vi "MC Control Loop.vi"() -> ()   [LabVIEW 2014]
uses:
  MC State Machine.lvsc/StatechartState.ctl
  MC State Machine.lvsc/State.ctl
  CAN Frame.ctl
  <vilib>/Platform/TimedLoop/XDataNode/timing_clust.ctl
  <vilib>/Platform/TimedLoop/XDataNode/nitl_modes.ctl
  <vilib>/Platform/TimedLoop/XDataNode/wakeup.ctl
  Remote Calibration/Remote Calibration Typedef.ctl
  MC State Machine.lvsc/Inputs.ctl
  AIR Status.ctl
  MC State Machine.lvsc/CompanionDiagram.vi/6/SC Main.vi
  CAN/8byte to 4 2byte.vi
  CAN/Decode VSM.vi
  CAN/Decode Inverter State.vi
  CAN/Decode Inverter Enable States.vi
  CAN/Decode Inverter Command Modes.vi
  CAN/MC/Process Run Fault.vi
  CAN/BMS/Decode Car State.vi
  CAN/BMS/Scale Cell Voltage.vi
  CAN/BMS/Scale Cell Temp.vi
  MC State Machine.lvsc/CompanionDiagram.vi/6/Upd State.vi
  MC State Machine.lvsc/CompanionDiagram.vi/6/Trans Graph0.vi
  MC State Machine.lvsc/CompanionDiagram.vi/6/EnterGraphCore.vi
  CAN/Send Throttle Signal.vi
  CAN/Disable Controller.vi
  CAN/MC/Clear Faults.vi
  CAN/Init Controller.vi
  CAN/MC/Send Parameter Message.vi
  <vilib>/FPGAPlugInAG/sbRIO-9626/niLvFpga_Open_sbRIO-9626.vi
  Global Data.vi
  <vilib>/Utility/error.llb/Error Cluster From Error Code.vi
  <vilib>/rvi/errors/niLvFpgaAdjustHostInterfaceError.vi
  MC State Machine.lvsc/CompanionDiagram.vi
  Percent to Torque Request.vi
  <vilib>/RioEmbeddedCAN/RioEmbeddedCAN.llb/CANWrite.vi
  <vilib>/FPGAPlugInAG/sbRIO-9626/niLvFpga_Close_sbRIO-9626.vi
  CAN/BMS/Decode Charging State.vi
  <vilib>/rvi/interface/nirviOpenFPGA/nirviOpenFPGA.xnode
  FPGA Bitfiles/FormulaElectric2_FPGATarget_FPGA_8a5J0mMac2U.lvbitx
  <vilib>/Platform/TimedLoop/XDataNode/XDataNode.xnode
  MC State Machine.lvsc/Trigger.ctl
  <vilib>/rvi/interface/nirviReadWriteControl/nirviReadWriteControl.xnode
  <vilib>/Statechart/Infrastructure/RTStatechart/RunTime SCN.xnode
  MC State Machine.lvsc/Outputs.ctl
  MC State Machine.lvsc
  <vilib>/rvi/interface/nirviCloseFPGA/nirviCloseFPGA.xnode
  <vilib>/Platform/TimedLoop/XDataNode/XDNodeRunTimeDep.lvlib
  NiFpgaLv.dll
panel:
  in  "Adjust Gamma Offset":bool
  in  "Gamma Adjust":dbl=120.0
  out "Active States":T1=[enum."Disabled"]
  in  "MC Update Period (ms)":u32=100
  in  "Zero Torque %":dbl
  in  "MC CAN Offset":u32=512 format="%x"
  in  "Regen Mult.":dbl
  in  "Torque Mult.":dbl=160.0
  in  "Activation Brake Pressure":dbl=50.0
  out "Torque Request":dbl=nan
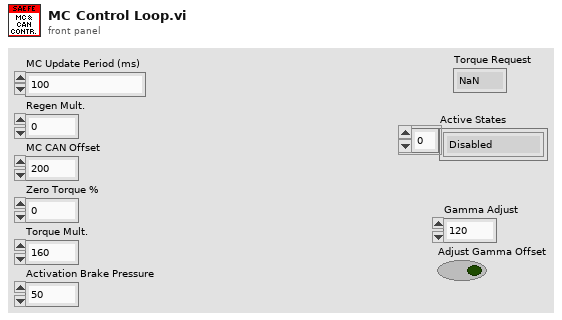
[diagram p1: front panel]
types:
  T1 = typedef "MC State Machine.lvsc/StatechartState.ctl" = T2[]
  T2 = typedef "MC State Machine.lvsc/State.ctl" = enum16{"NI.SC.Initial", "NI.SC.History", "NI.SC.ShallowHistory", "NI.SC.Terminal", "Let Current Drop then Disable AIR's", "Enabled", "Disabled"}
  T3 = typedef "CAN Frame.ctl" = cluster{"Time Stamp":timestamp, "Identifier":u32, "Extended":bool, "type":u8, "Payload":u8, "Payload 2":u8, "Payload 3":u8, "Payload 4":u8, "Payload 5":u8, "Payload 6":u8, "Payload 7":u8, "Payload 8":u8}
  T4 = cluster{"read mode":enum16{"polling", "blocking"}, "write mode":enum16{"polling", "blocking"}}
  T5 = typedef "Remote Calibration Typedef.ctl" = cluster{"Rear BP Scaling Factor":fxp<+,11,11>, "Front BP Scaling Factor":fxp<+,11,11>, "Rear BP Offset (V)":fxp<+/-,26,5>, "Front BP Offset":fxp<+/-,26,5>, "Throttle 2 Max":fxp<+,16,4>, "Throttle 2 Min":fxp<+,16,4>, "Throttle 1 Max":fxp<+,16,4>, "Throttle 1 Min":fxp<+,16,4>, "MC Update Period (ms)":u32, "Regen Mult.":dbl, "Zero Torque %":dbl, "Torque Mult.":dbl, "Activation Brake Pressure":dbl}
  T6 = typedef "XDNodeRunTimeDep.lvlib/timing_clust.ctl" = cluster{"Expected End [f-1]":u64, "Actual End [f-1]":u64, "Finished Late? [f-1]":bool, "Expected End [i-1]":u64, "Actual End [i-1]":u64, "Finished Late? [i-1]":bool, "Expected Start [i]":u64, "Actual Start [i]":u64, "Expected Start [f]":u64, "Actual Start [f]":u64, "Source Name":string, "Structure Name":string, "Period":i64, "Deadline":i64, "Offset":i64, "Start":i64, "Priority":i32, "Timeout":i32, "Mode":T7, "Wakeup Reason":T8, "Error":errorcluster, "Source Type":string, "Secondary Source Type":string, "Global End Time":u64, "Global Start Time":u64, "Frame Duration":u64, "Iteration Duration":u64, "Assigned CPU":i32, "I/O Scan Engine Mode":u32}
  T7 = typedef "XDNodeRunTimeDep.lvlib/nitl_modes.ctl" = enum32{"No Change", "Process missed periods, maintain original phase", "Discard missed periods, maintain original phase", "Process missed periods, ignore original phase", "Discard missed periods, ignore original phase"}
  T8 = typedef "XDNodeRunTimeDep.lvlib/wakeup.ctl" = enum32{"Normal", "Aborted", "Asynchronous wakeup", "Timing source error", "Timed loop error", "Timeout"}
  T9 = typedef "MC State Machine.lvsc/Inputs.ctl" = cluster{"Zero Torque %":dbl, "CAN Offset":u32, "Torque Mult.":dbl, "Regen Mult.":dbl, "Activation Brake Pressure":dbl, "stop":bool, "Average Throttle %":dbl, "Front Brake Pressure (psi)":dbl, "Motor Controller Dash Switch":bool, "Throttles OK?":bool, "AIR Status":T10, "CAN error":errorcluster, "CAN in":refnum<k20>, "tdms file":refnum<k34>, "tdms error":errorcluster, "Sampling Frequency (Hz)":dbl}
  T10 = typedef "AIR Status.ctl" = enum16{"Off", "Precharge", "On"}
  T11 = typedef "MC State Machine.lvsc/Outputs.ctl" = cluster{"Torque Request":dbl, "CAN error":errorcluster, "CAN out":refnum<k20>, "tdms file":refnum<k34>, "tdms error":errorcluster}
  T12 = typedef "CANFrameControl.ctl" = cluster{"identifier":u32, "extended?":bool, "type":u8, "payload":u8[]}
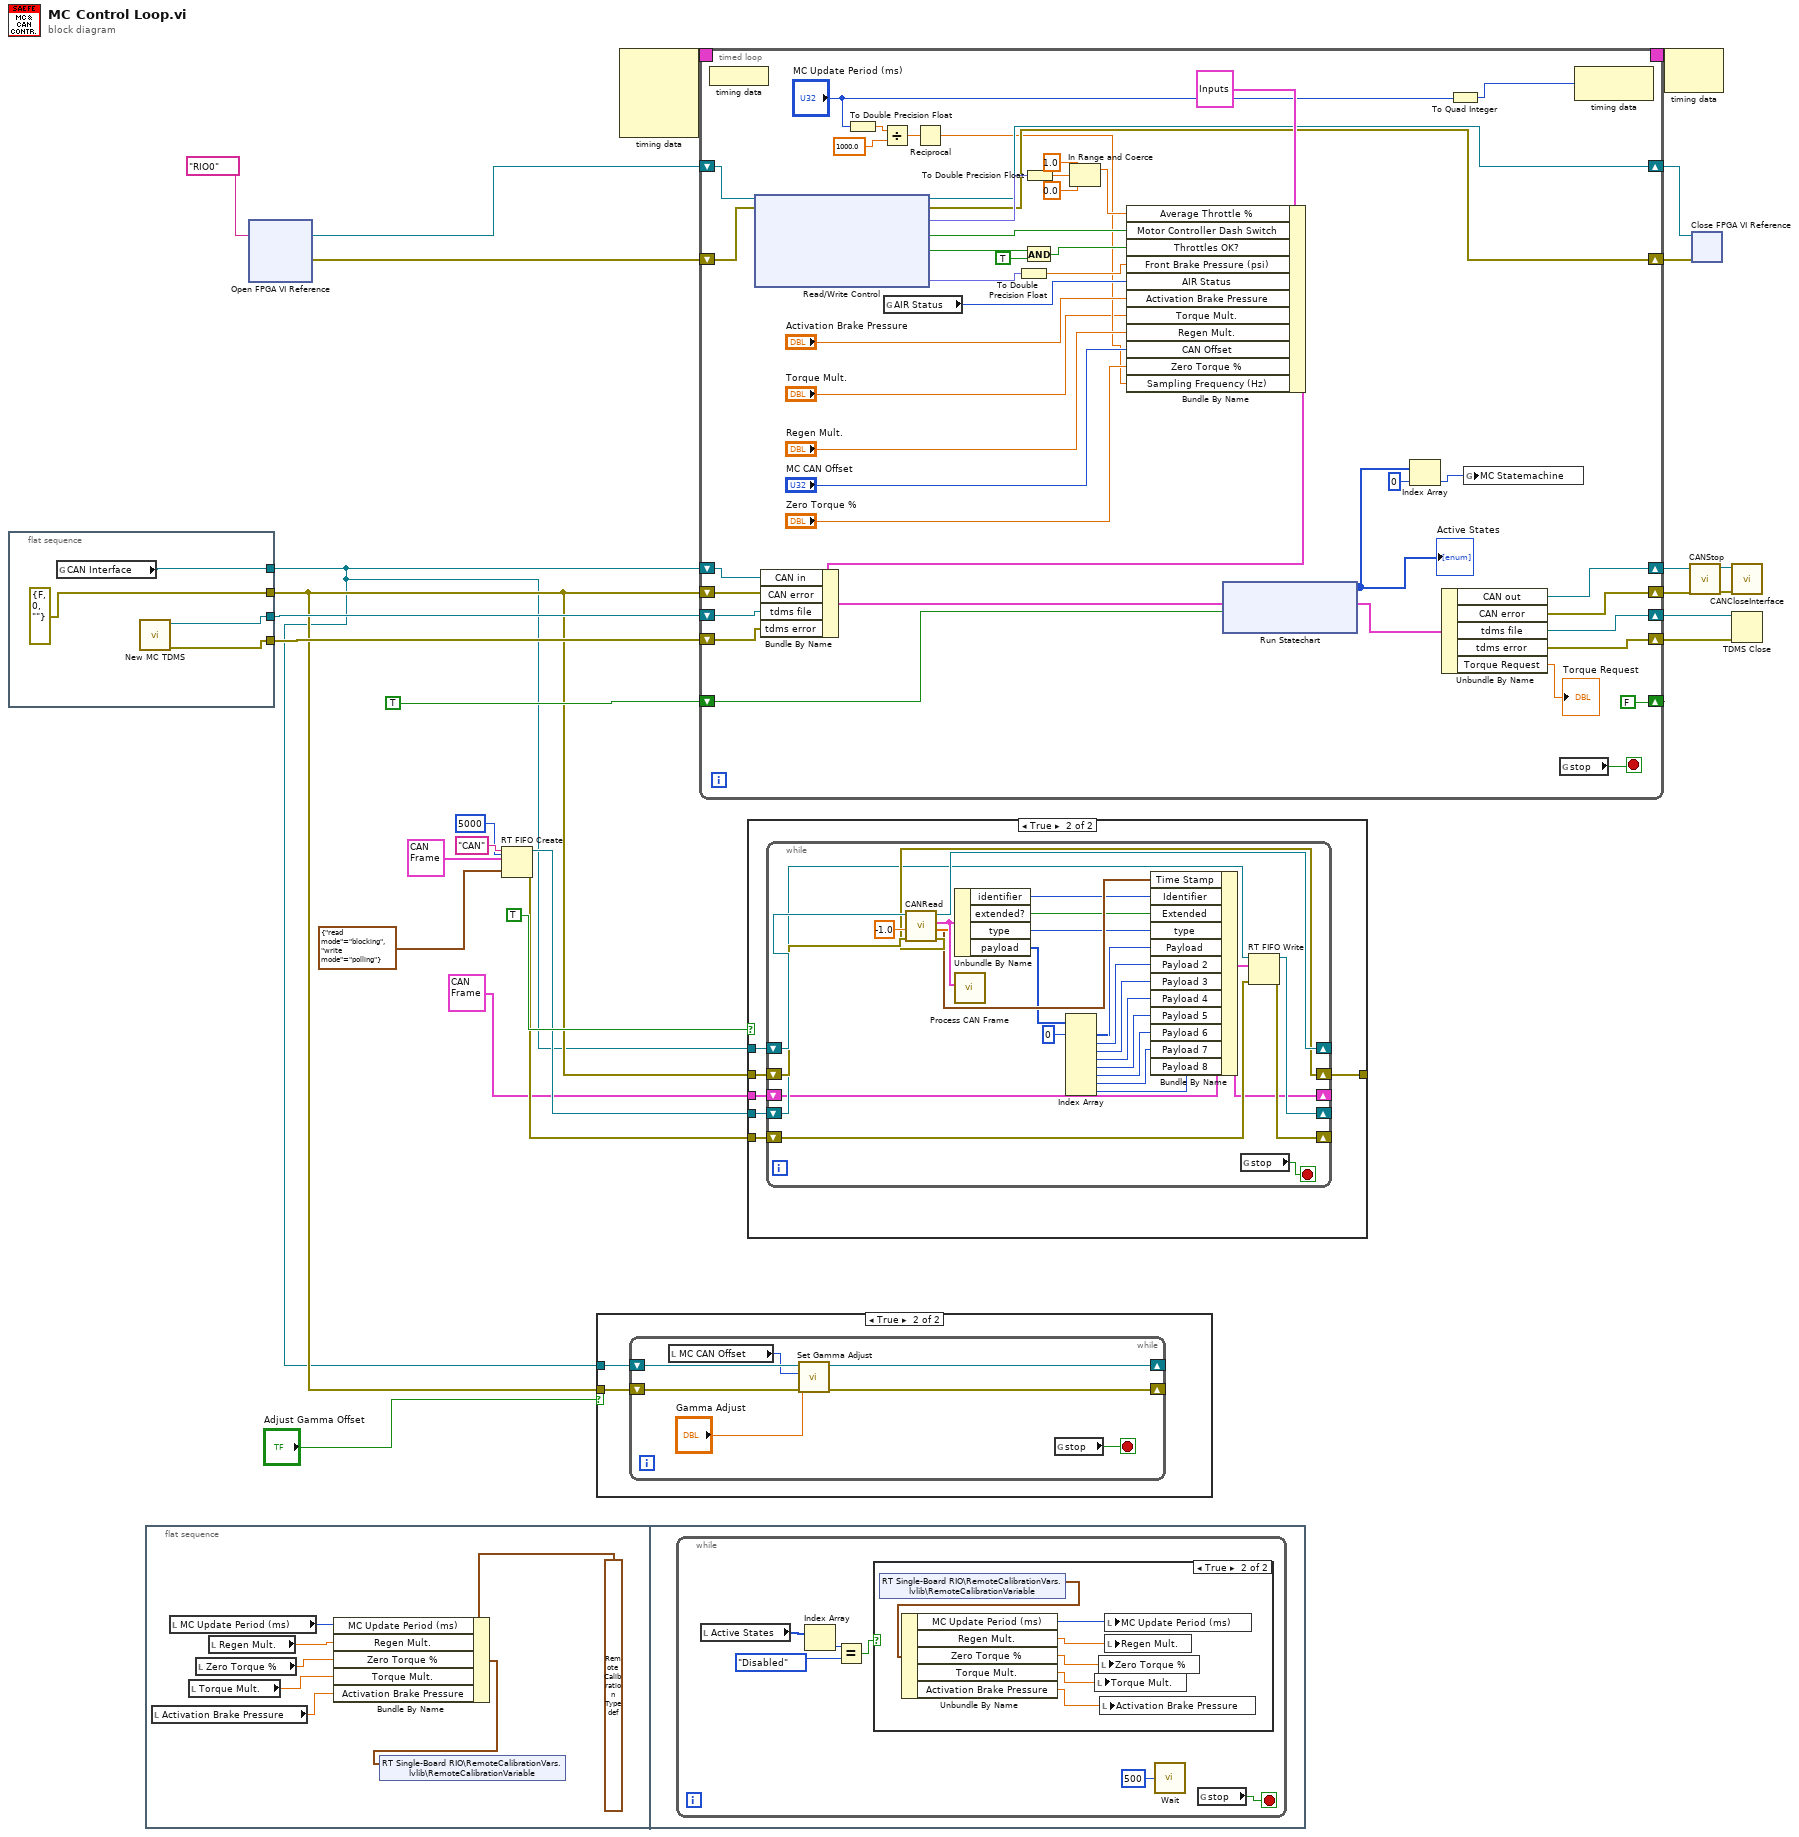
[diagram p0: block diagram]
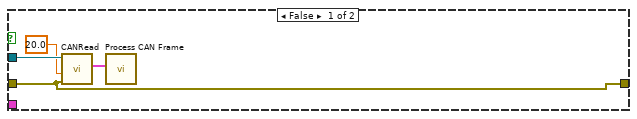
[diagram p4: hidden frame]
diagram:
  n1 = flat-sequence {
    tunnel: [errorcluster {"status"=FALSE, "code"=0, "source"=""} ("error out")] -> w2
    tunnel: [w28] -> w1
    tunnel: [w31] -> w5
    tunnel: [w30] -> w14
    frame #0 {
      n2 = global read "Global Data.vi" "CAN Interface"() -> (w28:refnum<k20>)
      n3 = call "New MC TDMS.vi"() -> ("error out"=w30:errorcluster, "Refnum out"=w31:refnum<k34>)  [unwired: 10 in]
    }
  }
  n4 = flat-sequence {
    frame #0 {
      n5 = local read "Activation Brake Pressure"() -> (w33:dbl)
      n6 = local read "MC Update Period (ms)"() -> (w37:u32)
      n7 = local read "Torque Mult."() -> (w34:dbl)
      n8 = local read "Zero Torque %"() -> (w35:dbl)
      n9 = local read "Regen Mult."() -> (w36:dbl)
      n10 = Bundle By Name(cluster=T5 {"Rear BP Scaling Factor"=1250.0, "Front BP Scaling Factor"=1250.0, "Rear BP Offset (V)"=0.4820899963378906, "Front BP Offset"=0.4808177947998047, "Throttle 2 Max"=3.89990234375, "Throttle 2 Min"=2.090087890625, "Throttle 1 Max"=0.6298828125, "Throttle 1 Min"=2.4599609375, "MC Update Period (ms)"=20, "Regen Mult."=0.0, "Zero Torque %"=0.0, "Torque Mult."=160.0, "Activation Brake Pressure"=50.0} ("RemoteCalibrationVariable"), "MC Update Period (ms)"=w37, "Regen Mult."=w36, "Zero Torque %"=w35, "Torque Mult."=w34, "Activation Brake Pressure"=w33) -> (w32:T5)
      n11 = shared-variable "RT Single-Board RIO\\RemoteCalibrationVars.lvlib\\RemoteCalibrationVariable"(w32) -> ()  [unwired: 1 in, 1 out]
    }
    frame #1 {
      n12 = while {
        stop <- w43 stop-if-true
        n13 = local read "Active States"() -> (w42:T1)
        n14 = Index Array(array=w42) -> (element=w41:T2)  [unwired: 1 in]
        n15 = Equal?(x=w41, y=State."Disabled") -> (x = y?=w40:bool)
        n16 = case shown="True" w40 {
          frame False {
          }
          frame True {
            n17 = shared-variable "RT Single-Board RIO\\RemoteCalibrationVars.lvlib\\RemoteCalibrationVariable"() -> (w50:T5)  [unwired: 1 in, 1 out]
            n18 = Unbundle By Name(w50) -> ("MC Update Period (ms)"=w49:u32, "Regen Mult."=w48:dbl, "Zero Torque %"=w47:dbl, "Torque Mult."=w46:dbl, "Activation Brake Pressure"=w45:dbl)
            n19 = local write "Torque Mult."(w46) -> ()
            n20 = local write "Zero Torque %"(w47) -> ()
            n21 = local write "Activation Brake Pressure"(w45) -> ()
            n22 = local write "MC Update Period (ms)"(w49) -> ()
            n23 = local write "Regen Mult."(w48) -> ()
          }
        }
        n24 = call "Wait"("Count(mSec)"=u32 500) -> ()  [unwired: 1 out]
        n25 = global read "Global Data.vi" "stop"() -> (w43:bool)
      }
    }
  }
  n26 = xnode "Open FPGA VI Reference"("resource name"=tag "RIO0") -> ("FPGA VI Reference Out"=w16:refnum<k20>, "error out"=w15:errorcluster)  [unwired: 1 in]
  n27 = RT FIFO Create(0:"CAN" ("name (unnamed)"), 1:T3 {"Time Stamp"=timestamp(0 s since 1904-01-01), "Identifier"=0, "Extended"=FALSE, "type"=0, "Payload"=0, "Payload 2"=0, "Payload 3"=0, "Payload 4"=0, "Payload 5"=0, "Payload 6"=0, "Payload 7"=0, "Payload 8"=0} ("CAN Frame"), 4:u32 5000 ("size (10)"), 7:T4 {"read mode"=enum."blocking", "write mode"=enum."polling"} ("r/w modes (polling,polling)")) -> (8:w11:refnum<k33>, 11:w10:errorcluster)  [unwired: 4 in, 1 out]
  n28 = case shown="True" "Adjust Gamma Offset" {
    tunnel: w2 -> [_ w52]
    tunnel: w1 -> [_ w51]
    frame False {
    }
    frame True {
      n29 = while {
        shift-right: [w53] -> _
        shift-left: w52 -> [w58]
        shift-right: [w54] -> _
        shift-left: w51 -> [w57]
        stop <- w59 stop-if-true
        n30 = local read "MC CAN Offset"() -> (w56:u32)
        n31 = call "Set Gamma Adjust.vi"("error in (no error)"=w58, "Gamma Adjust"="Gamma Adjust", "CAN Offset"=w56, "interface object in"=w57) -> ("error out"=w53:errorcluster, "interface object out"=w54:refnum<k20>)  [unwired: 6 in]
        n32 = global read "Global Data.vi" "stop"() -> (w59:bool)
      }
    }
  }
  n33 = node-c288() -> (w19:T6)  [unwired: 4 in]
  n34 = timed-loop {
    shift-right: [w78] -> w27
    shift-left: w2 -> [w90]
    shift-right: [w79] -> w26
    shift-left: w1 -> [w91]
    shift-right: [w84] -> w22
    shift-left: w15 -> [w105]
    shift-right: [w85] -> w23
    shift-left: w16 -> [w104]
    shift-right: [w77] -> w21
    shift-left: w5 -> [w89]
    shift-right: [w76] -> w9
    shift-left: w14 -> [w88]
    shift-right: [FALSE] -> _
    shift-left: TRUE -> [w83]
    timing: w19 -> [_]
    timing-out: [_] -> w18
    stop <- w80 stop-if-true
    n35 = node-c288() -> ()  [unwired: 1 in]
    n36 = xnode "Read/Write Control"("FPGA VI Reference In"=w104, "error in"=w105) -> ("FPGA VI Reference Out"=w85:refnum<k20>, "error out"=w84:errorcluster, "Average Throttle (%)"=w101:fxp<+/-,33,22>, "Motor Controller Dash Switch"=w74:bool, "Throttles In Range?"=w100:bool, "Rear BP (psi)"=w98:fxp<+,26,13>)  [unwired: 1 out]
    n37 = To Double Precision Float(number="MC Update Period (ms)") -> (double precision float=w65:dbl)
    n38 = Divide(x=w65, y=1000.0) -> (x/y=w63:dbl)
    n39 = global read "Global Data.vi" "AIR Status"() -> (w97:T10)
    n40 = Reciprocal(x=w63) -> (1/x=w62:dbl)
    n41 = To Double Precision Float(number=w98) -> (double precision float=w99:dbl)
    n42 = And(x=w100, y=TRUE) -> (x .and. y?=w75:bool)
    n43 = To Double Precision Float(number=w101) -> (double precision float=w70:dbl)
    n44 = In Range and Coerce(upper limit=1.0, x=w70, lower limit=0.0) -> (coerced(x)=w67:dbl)  [unwired: 1 out]
    n45 = Bundle By Name(cluster=T9 {"Zero Torque %"=15.0, "CAN Offset"=160, "Torque Mult."=2.4, "Regen Mult."=0.5, "Activation Brake Pressure"=100.0, "stop"=FALSE, "Average Throttle %"=0.0, "Front Brake Pressure (psi)"=0.0, "Motor Controller Dash Switch"=FALSE, "Throttles OK?"=FALSE, "AIR Status"=enum."Off", "CAN error"={"status"=FALSE, "code"=0, "source"=""}, "CAN in"=refnum, "tdms file"=refnum, "tdms error"={"status"=FALSE, "code"=0, "source"=""}, "Sampling Frequency (Hz)"=0.0} ("Inputs"), "Average Throttle %"=w67, "Motor Controller Dash Switch"=w74, "Throttles OK?"=w75, "Front Brake Pressure (psi)"=w99, "AIR Status"=w97, "Activation Brake Pressure"="Activation Brake Pressure", "Torque Mult."="Torque Mult.", "Regen Mult."="Regen Mult.", "CAN Offset"="MC CAN Offset", "Zero Torque %"="Zero Torque %", "Sampling Frequency (Hz)"=w62) -> (w92:T9)
    n46 = Bundle By Name(cluster=w92, "CAN in"=w91, "CAN error"=w90, "tdms file"=w89, "tdms error"=w88) -> (w87:T9)
    n47 = xnode "Run Statechart"("Init?"=w83, "Inputs"=w87) -> ("Outputs"=w103:T11, "Active States"=w73:T1)  [unwired: 1 in, 1 out]
    "Active States" <- w73
    n48 = Index Array(array=w73, index=0) -> (element=w71:T2)
    n49 = Unbundle By Name(w103) -> ("CAN out"=w79:refnum<k20>, "CAN error"=w78:errorcluster, "tdms file"=w77:refnum<k34>, "tdms error"=w76:errorcluster, "Torque Request"=→"Torque Request":dbl)
    n50 = To Quad Integer(1:"MC Update Period (ms)") -> (0:w81:i64)
    n51 = global write "Global Data.vi" "MC Statemachine"(w71) -> ()
    n52 = global read "Global Data.vi" "stop"() -> (w80:bool)
    n53 = node-c288(w81) -> ()  [unwired: 1 out]
  }
  n54 = case shown="True" TRUE {
    tunnel: w1 -> [w144 w150]
    tunnel: w2 -> [w143 w149]
    tunnel: [w143 w148] -> _
    tunnel: w11 -> [_ w147]
    tunnel: w10 -> [_ w146]
    tunnel: T3 {"Time Stamp"=timestamp(0 s since 1904-01-01), "Identifier"=0, "Extended"=FALSE, "type"=0, "Payload"=0, "Payload 2"=0, "Payload 3"=0, "Payload 4"=0, "Payload 5"=0, "Payload 6"=0, "Payload 7"=0, "Payload 8"=0} ("CAN Frame") -> [_ w145]
    frame False {
      n55 = call <vilib>:"CANRead.vi"("error in (no error)"=w143, "timeout (0 s)"=20.0, "interface object in"=w144) -> ("CAN frame"=w141:T12)  [unwired: 5 in, 3 out]
      n56 = call "Process CAN Frame.vi"("CAN frame"=w141) -> ()  [unwired: 11 in]
    }
    frame True {
      n57 = while {
        shift-right: [w177] -> _
        shift-left: w150 -> [w176]
        shift-right: [w173] -> w148
        shift-left: w149 -> [w174]
        shift-right: [w164] -> _
        shift-left: w147 -> [w167]
        shift-right: [w165] -> _
        shift-left: w146 -> [w166]
        shift-right: [w161] -> _
        shift-left: w145 -> [w162]
        stop <- w172 stop-if-true
        n58 = call <vilib>:"CANRead.vi"("error in (no error)"=w174, "timeout (0 s)"=-1.0, "interface object in"=w176) -> ("error out"=w173:errorcluster, "timestamp"=w171:timestamp, "CAN frame"=w163:T12, "interface object out"=w177:refnum<k20>)  [unwired: 5 in]
        n59 = Unbundle By Name(w163) -> ("identifier"=w170:u32, "extended?"=w169:bool, "type"=w168:u8, "payload"=w160:u8[])
        n60 = call "Process CAN Frame.vi"("CAN frame"=w163) -> ()  [unwired: 11 in]
        n61 = Index Array(array=w160, index #1=0 ("index")) -> (element #1=w158:u8, element #2=w157:u8, element #3=w156:u8, element #4=w155:u8, element #5=w154:u8, element #6=w153:u8, element #7=w152:u8, element #8=w151:u8)  [unwired: 7 in]
        n62 = Bundle By Name(cluster=w162, "Time Stamp"=w171, "Identifier"=w170, "Extended"=w169, "type"=w168, "Payload"=w158, "Payload 2"=w157, "Payload 3"=w156, "Payload 4"=w155, "Payload 5"=w154, "Payload 6"=w153, "Payload 7"=w152, "Payload 8"=w151) -> (w161:T3)
        n63 = global read "Global Data.vi" "stop"() -> (w172:bool)
        n64 = RT FIFO Write(0:w167, 1:w161, 3:w166) -> (8:w164:refnum<k33>, 11:w165:errorcluster)  [unwired: 2 in, 2 out]
      }
    }
  }
  n65 = node-c288(w18) -> ()  [unwired: 1 out]
  n66 = call <vilib>:"CANStop.vi"("error in (no error)"=w27, "interface object in"=w26) -> ("error out"=w25:errorcluster, "interface object out"=w24:refnum<k20>)  [unwired: 8 in]
  n67 = xnode "Close FPGA VI Reference"("FPGA VI Reference In"=w23, "error in"=w22) -> ()  [unwired: 1 out]
  n68 = call <vilib>:"CANCloseInterface.vi"("error in (no error)"=w25, "interface object in"=w24) -> ()  [unwired: 9 in, 1 out]
  n69 = TDMS Close(8:w9, 11:w21) -> ()  [unwired: 2 out]
